vi "set tuner gain mode.vi"(8 "error in (no error)":errorcluster, 10 "AutoGain":bool, 11 "DeviceRefnum":u64) -> (0 "error out":errorcluster, 2 "function return":i32, 3 "DeviceRefnum Out":u64)   [LabVIEW 2015, in "rtlsdr.lvlib"]
doc: "Set the gain mode (automatic/manual) for the device. Manual gain mode must be enabled for the gain setter function to work."
uses:
  rtlsdr.lvlib
  rtlsdr/rtlsdr.dll
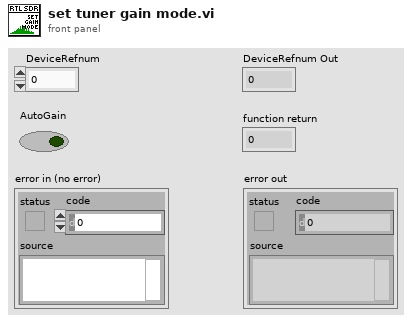
[diagram p1: front panel]
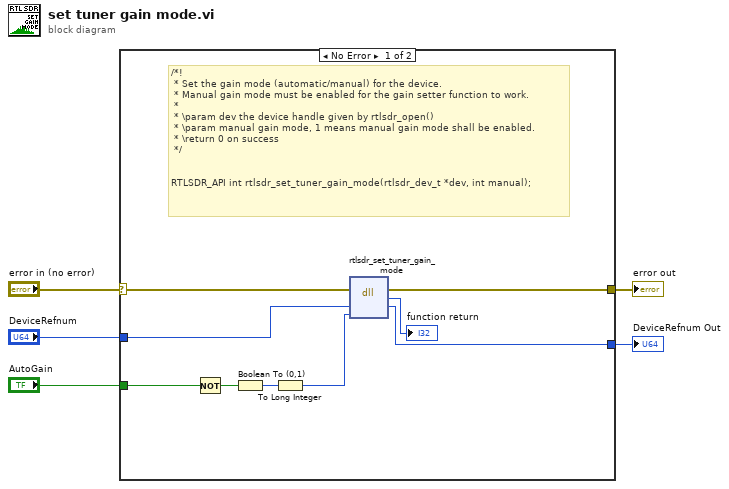
[diagram p0: block diagram]
diagram:
  n1 = case shown="No Error" "error in (no error)" {
    selector: "error in (no error)" -> [w6 w16]
    tunnel: [w13 w16] -> w5
    tunnel: "DeviceRefnum" -> [w12 w15]
    tunnel: [w11 w15] -> w3
    tunnel: "AutoGain" -> [w10 _]
    frame No Error {
      # "/*!\n * Set the gain mode (automatic/manual) for the device.\n * Manual gain mode must be enabled for the gain setter function to work.\n *\n * \\param dev the device handle given by rtlsdr_open()\n * \\param manual gain mode, 1 means manual gain mode shall be enabled.\n * \\return 0 on success\n */\n\n\nRTLSDR_API int rtlsdr_set_tuner_gain_mode(rtlsdr_dev_t *dev, int manual);"
      n2 = Not(x=w10) -> (.not. x?=w9:bool)
      n3 = Boolean To (0,1)(Boolean=w9) -> (0, 1=w8:i16)
      n4 = To Long Integer(number=w8) -> (32bit integer=w7:i32)
      n5 = dll-call lib="C:/Users/TheDoctor/Documents/Projects/Labview Libraries/rtlsdr/rtlsdr.*" fn="rtlsdr_set_tuner_gain_mode"(error in=w6, "DeviceRefnum"=w12, "GainMode"=w7) -> (error out=w13:errorcluster, "return type"=→"function return":i32, "DeviceRefnum"=w11:u64)  [unwired: 3 in, 1 out]
    }
    frame Error {
    }
  }
  "error out" <- w5
  "DeviceRefnum Out" <- w3
